vi "Set ABORT Color.vi"(8 "error in (no error)":errorcluster, 11 "Common GUI v3 in":refnum<class "Common GUI v3.lvclass">) -> (0 "error out":errorcluster, 3 "Common GUI v3 out":refnum<class "Common GUI v3.lvclass">)   [LabVIEW 2026, in "TALOS.lvlib" / "Common GUI v3.lvlib" / "Common GUI v3.lvclass"]
uses:
  Common GUI v3.lvclass
  Ancestor/Ancestor/Ancestor.lvclass/Ancestor.ctl
  Common GUI v3.lvclass/Common GUI v3.ctl
  Support VIs/Generate Error.vi
  FGV/Error Memory/Get Error Description.vi
  Support VIs/Get PC name.vi
  Ancestor/Ancestor/Read ID.vi
  Support VIs/Get Class Name.vi
  <vilib>/Utility/error.llb/Clear Errors.vi
  FGV/Error Memory/Error Memory Core.vi
  <vilib>/AdvancedString/Delimited String to 1D String Array.vi
  <vilib>/AdvancedString/Delimited String to 1D String Array (string).vi
  Support VIs/Circus Root Path.vi
  FGV/Error Memory/Error Crt Lvl checker.vi
  FGV/Error Memory/Error Memory Core.vi/40c8088d-b597-4017-91af-faa98e00292e.vi
  FGV/Error Memory/Error Memory Core.vi/d4a3ab98-063c-4e44-b43d-fbdcfe6c2be2.vi
  Support VIs/Global Memory.vi
  <vilib>/Utility/LVClass/Get LV Class Name.vi
  Support VIs/Is in Packed Library.vi
  Support VIs/TALOS Root path.vi
  Support VIs/Read CSV worksheet.vi
  Support VIs/Global Constants.vi
  <vilib>/Utility/error.llb/General Error Handler.vi
  <vilib>/Utility/config.llb/Open Config Data.vi
  <vilib>/Utility/config.llb/Get Section Names.vi
  <vilib>/Utility/config.llb/Get Key Names.vi
  <vilib>/Utility/config.llb/Read Key.vi
  <vilib>/Utility/config.llb/Read Key (String).vi
  <vilib>/Utility/config.llb/Close Config Data.vi
  Support VIs/Error Log.vi
  Ancestor/Ancestor/Ancestor.lvclass
  <vilib>/Comparison/Equal/Equal Functor/Equal Functor.lvclass
  TALOS.lvlib
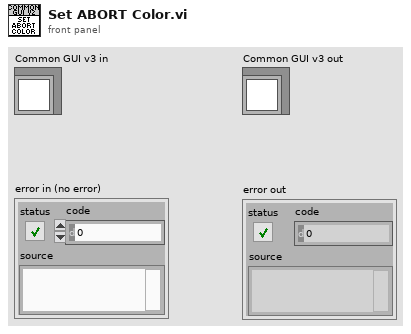
[diagram p1: front panel]
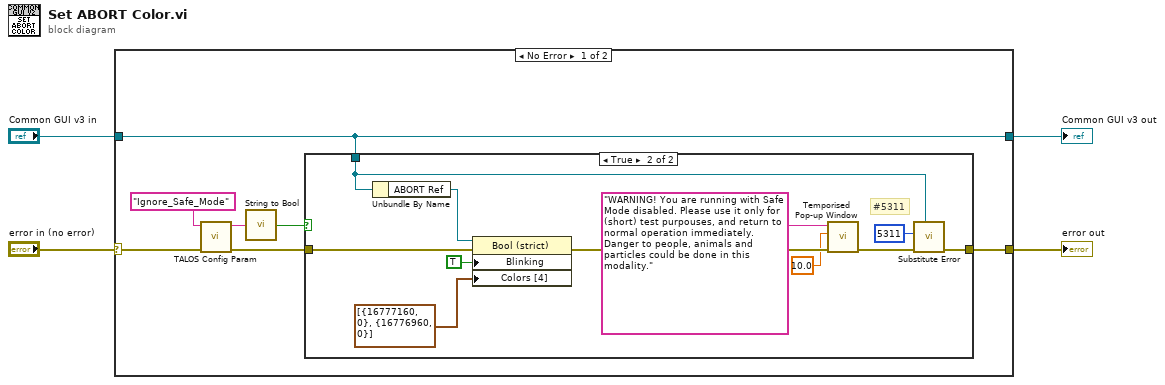
[diagram p0: block diagram]
diagram:
  n1 = case shown="No Error" "error in (no error)" {
    selector: "error in (no error)" -> [w9 w25]
    tunnel: "Common GUI v3 in" -> [w11 w24]
    tunnel: [w5 w25] -> w2
    tunnel: [w11 w24] -> w1
    frame No Error {
      n2 = call "TALOS Config Param.vi"("error in (no error)"=w9, "Parameter Name"="Ignore_Safe_Mode") -> ("error out"=w6:errorcluster, "Output"=w8:string)  [unwired: 8 in]
      n3 = call "String to Bool.vi"("String"=w8) -> ("Boolean"=w7:bool)
      n4 = case shown="True" w7 {
        tunnel: w11 -> [_ w15]
        tunnel: w6 -> [w12 w20]
        tunnel: [w12 w16] -> w5
        frame False {
        }
        frame True {
          # "#5311"
          n5 = Unbundle By Name(w15) -> ("ABORT Ref"=w23:refnum<vi>)
          n6 = property class="Bool (strict)"(reference=w23, error in=w20, "Blinking"=TRUE, "Colors [4]"=cluster{u32, u32}[] [{16777160, 0}, {16776960, 0}] ("Colors")) -> (error out=w19:errorcluster)  [unwired: 1 out]
          n7 = call "Temporised Pop-up Window.vi"("error in (no error)"=w19, "Timeout"=10.0, "Text"="WARNING! You are running with Safe Mode disabled. Please use it only for (short) test purpouses, and return to normal operation immediately. Danger to people, animals and particles could be done in this modality.") -> ("error out"=w17:errorcluster)  [unwired: 8 in]
          n8 = call "Substitute Error.vi"("LabVIEW Object"=w15, "error in (no error)"=w17, "Error Code"=5311) -> ("error out"=w16:errorcluster)  [unwired: 8 in]
        }
      }
    }
    frame Error {
    }
  }
  "error out" <- w2
  "Common GUI v3 out" <- w1
